vi "set nonvolatile memory.vi"(8 "error in (no error)":errorcluster, 10 "nonvolatile_memory":T1, 11 "id":i32) -> (0 "error out":errorcluster, 3 "function return":i32)   [LabVIEW 2012, in "libximc.lvlib"]
doc: "result_t XIMC_API set_nonvolatile_memory (device_t id, const nonvolatile_memory_t* nonvolatile_memory);"
uses:
  libximc.lvlib
  libximc.dll
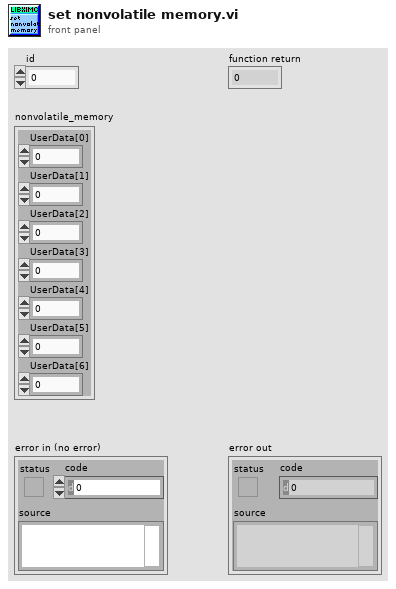
[diagram p1: front panel]
types:
  T1 = cluster{"UserData[0]":u32, "UserData[1]":u32, "UserData[2]":u32, "UserData[3]":u32, "UserData[4]":u32, "UserData[5]":u32, "UserData[6]":u32}
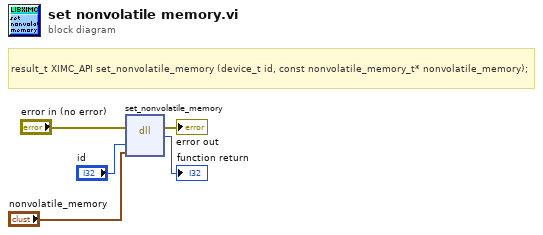
[diagram p0: block diagram]
diagram:
  # "result_t XIMC_API set_nonvolatile_memory (device_t id, const nonvolatile_memory_t* nonvolatile_memory);"
  n1 = dll-call lib="E:/labview-2.12.1-Labview_12.0/ximcLVx32/libximc.*" fn="set_nonvolatile_memory"(error in="error in (no error)", "id"="id", "nonvolatile_memory"="nonvolatile_memory") -> (error out=→"error out":errorcluster, →"function return":i32)  [unwired: 4 in, 1 out]
